vi "Subscriber.vi"() -> ()   [LabVIEW 2024]
uses:
  src/NATS Subscription/NATS Subscription.lvclass
  src/NATS Subscription/NATS Subscription.lvclass/NATS Subscription.ctl
  src/NATS Client/NATS Client.lvclass/NATS Client.ctl
  src/NATS Client/NATS Client.lvclass
panel:
  out "Unread Messages":i32
  out "Payload":string
  out "Received":timestamp format="%<%.0X %x>T"
  in  "Read":bool
  in  "Unsubscribe":bool
  out "Active Subscriptions":string[](array[string])
  in  "Query Active Subscriptions":bool
  out "error out":errorcluster
  out "loop error":errorcluster
  in  "Subscribe":bool
  in  "Subject":string="data.hello_world"
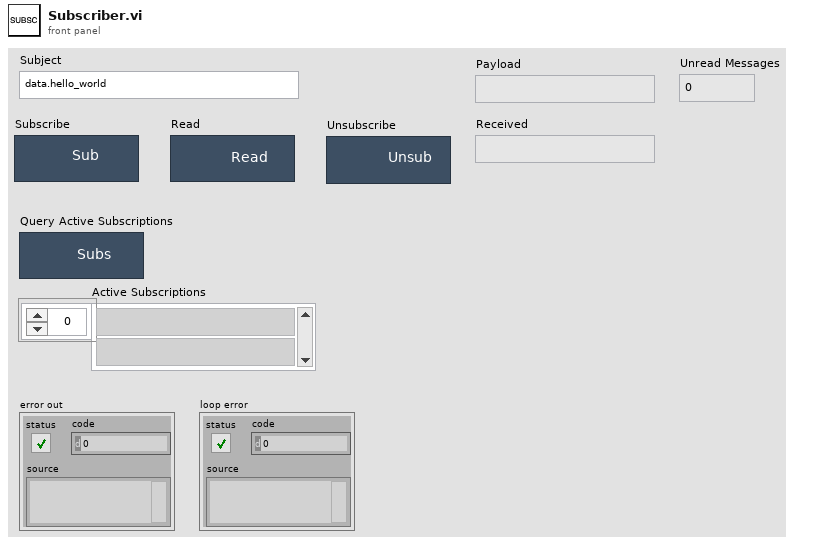
[diagram p1: front panel]
types:
  T1 = map{string, refnum<class "NATS Subscription.lvclass">}
  T2 = typedef "NATS Core.lvlib/nats message.ctl" = cluster{"subject":string, "payload":string, "sub id":string, "reply-to":string, "headers":string, "type":T3, "received":timestamp}
  T3 = typedef "NATS Core.lvlib/msg type.ctl" = enum16{"Undefined", "MSG", "HMSG", "+OK", "PING", "PONG", "-ERR", "INFO"}
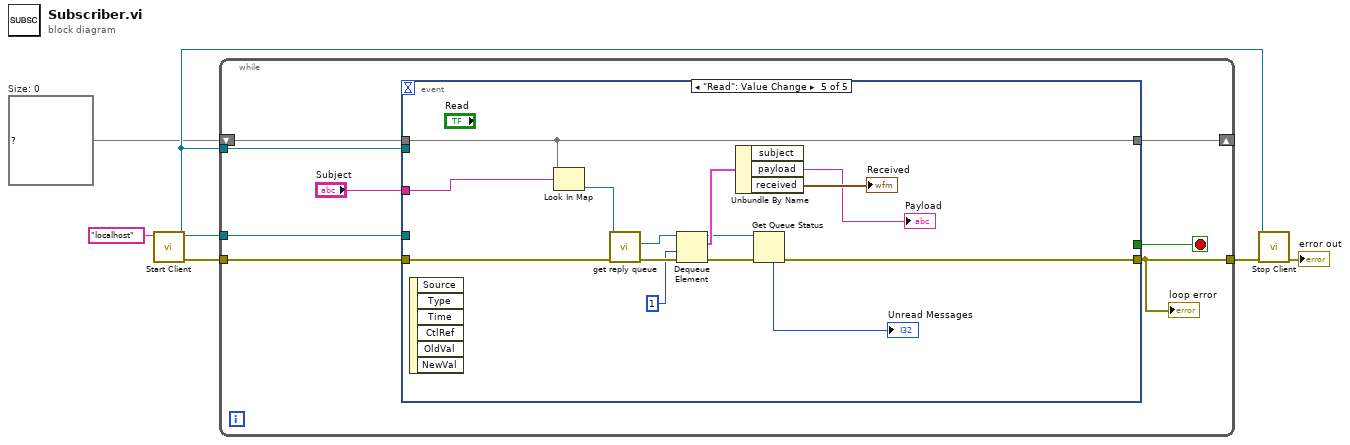
[diagram p0: block diagram]
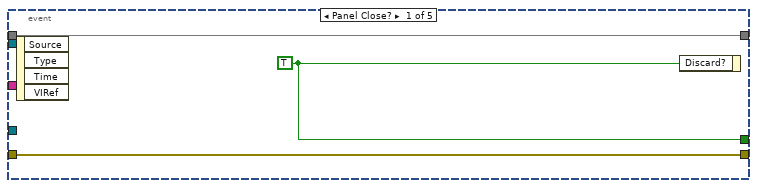
[diagram p2: hidden frame]
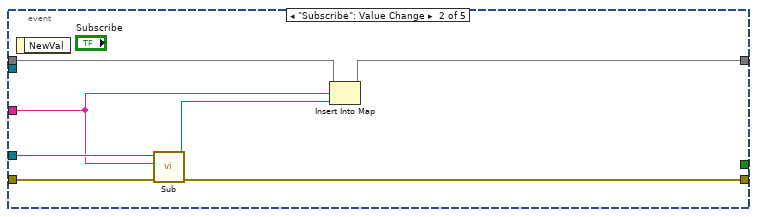
[diagram p3: hidden frame]
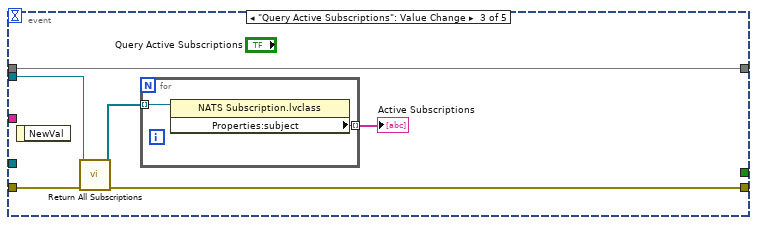
[diagram p4: hidden frame]
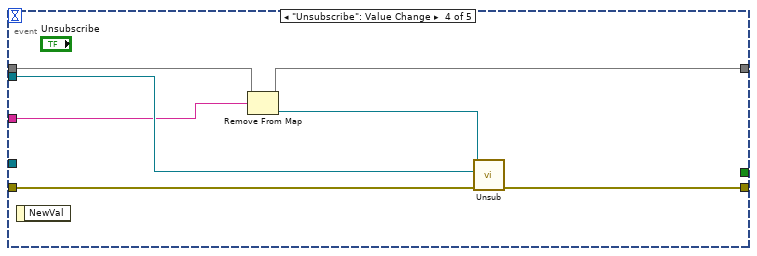
[diagram p5: hidden frame]
diagram:
  w1 = T1 {}  # Size: 0
  n1 = call "Start Client.vi"("address"="localhost") -> ("error out"=w6:errorcluster, "NATS Client out"=w3:refnum<class "NATS Client.lvclass">)  [unwired: 9 in]
  n2 = while {
    tunnel: w3 -> [w12]
    tunnel: w3 -> [w11]
    shift-right: [w10] -> _
    shift-left: w1 -> [w8]
    tunnel: w6 -> [w13]
    tunnel: [w9] -> w4
    stop <- w14 stop-if-true
    n3 = event shown="[4] \"Read\": Value Change" {
      selector: _ -> [_ _ _ _ _]
      dyn-events: _ -> [_ _ _ _ _]
      timeout: _ -> [_ _ _ _ _]
      tunnel: [w17 _ _ _ _] -> w14
      tunnel: w13 -> [w16 w23 w27 w37 w53]
      tunnel: [w16 w22 w26 w38 w42] -> w9
      tunnel: w12 -> [_ w24 _ _ _]
      tunnel: w11 -> [_ _ w28 w39 _]
      tunnel: [w15 w18 w25 w34 w46] -> w10
      tunnel: w8 -> [w15 w19 w25 w33 w46]
      tunnel: "Subject" -> [_ w21 _ w36 w52]
      event Panel Close? {
        w17 = TRUE ("Discard?")
        n4 = event-data() -> ()  [unwired: 1 in, 4 out]
        n5 = event-data("Discard?"=w17) -> ()  [unwired: 1 in, 1 out]
      }
      event "Subscribe": Value Change {
        n6 = event-data() -> ()  [unwired: 1 in, 1 out]
        n7 = call "Sub.vi"("error in"=w23, "subject"=w21, "NATS Client"=w24) -> ("error out"=w22:errorcluster, "NATS Subscription"=w20:refnum<class "NATS Subscription.lvclass">)  [unwired: 7 in]
        n8 = Insert Into Map(map in=w19, key=w21, value=w20) -> (map out=w18:T1)  [unwired: 2 out]
      }
      event "Query Active Subscriptions": Value Change {
        n9 = event-data() -> ()  [unwired: 1 in, 1 out]
        n10 = call "Return All Subscriptions.vi"("error in"=w27, "NATS Client"=w28) -> ("error out"=w26:errorcluster, "Subscriptions"=w30:refnum<class "NATS Subscription.lvclass">[])  [unwired: 8 in]
        n11 = for {
          tunnel: w30 -> [w32] mode=indexing
          tunnel: [w31] -> w29 mode=indexing
          n12 = property class="NATS Subscription.lvclass"(reference=w32) -> ("Properties:subject"=w31:string)  [unwired: 1 in, 2 out]
        }
        "Active Subscriptions" <- w29
      }
      event "Unsubscribe": Value Change {
        n13 = event-data() -> ()  [unwired: 1 in, 1 out]
        n14 = Remove From Map(10:w36, 11:w33) -> (1:w35:refnum<class "NATS Subscription.lvclass">, 3:w34:T1)  [unwired: 1 out]
        n15 = call "Unsub.vi"("error in"=w37, "NATS Client"=w39, "NATS Subscription"=w35) -> ("error out"=w38:errorcluster)  [unwired: 7 in, 1 out]
      }
      event "Read": Value Change {
        n16 = event-data() -> ()  [unwired: 1 in, 6 out]
        n17 = Look In Map(map=w46, key=w52) -> (value=w51:refnum<class "NATS Subscription.lvclass">)  [unwired: 1 in, 1 out]
        n18 = call "get reply queue.vi"("error in"=w53, "NATS Subscription in"=w51) -> ("error out"=w50:errorcluster, "reply queue"=w44:refnum<queue>)  [unwired: 7 in, 1 out]
        n19 = Dequeue Element(queue=w44, timeout in ms (-1)=1, error in (no error)=w50) -> (queue out=w41:refnum<queue>, element=w49:T2, error out=w43:errorcluster)  [unwired: 1 out]
        n20 = Unbundle By Name(w49) -> ("payload"=→"Payload":string, "received"=→"Received":timestamp)  [unwired: 1 out]
        n21 = Get Queue Status(queue=w41, error in (no error)=w43) -> (error out=w42:errorcluster, # elements in queue=→"Unread Messages":i32)  [unwired: 1 in, 6 out]
      }
    }
    "loop error" <- w9
  }
  n22 = call "Stop Client.vi"("error in"=w4, "NATS Client"=w3) -> ("error out"=→"error out":errorcluster)  [unwired: 9 in]
